vi "TalonSRXSetCoast.vi"(0 "Device Reference (in)":T1, 5 "Set Coast Mode":bool, 11 "Error (in)":errorcluster) -> (4 "Device Reference (out)":T1, 15 "Error (out)":errorcluster)   [LabVIEW 2020]
doc: "Wrapper for setting coast/brake mode for Talon SRX motor controllers."
uses:
  <vilib>/Rock Robotics/WPI/MotorControl/WPI_MotorControlDeviceRef.ctl
  <vilib>/Rock Robotics/WPI/MotorControl/WPI_MotorControlType.ctl
  <vilib>/Rock Robotics/SystemInterfaces/DIO/FPGA_DIOPWMChannel.ctl
  <vilib>/Rock Robotics/WPI/PWM/WPI_PWMDeadband.ctl
  <vilib>/Rock Robotics/SystemInterfaces/DIO/FPGA_DIOChannel.ctl
  <vilib>/Rock Robotics/WPI/ThirdParty/Phoenix-LabVIEW/Motor Controller/Controls/CTRE_Phoenix_MotorControl_NeutralMode.ctl
  3ee01901-79ae-4aa6-af32-efcf4cf19248.vi
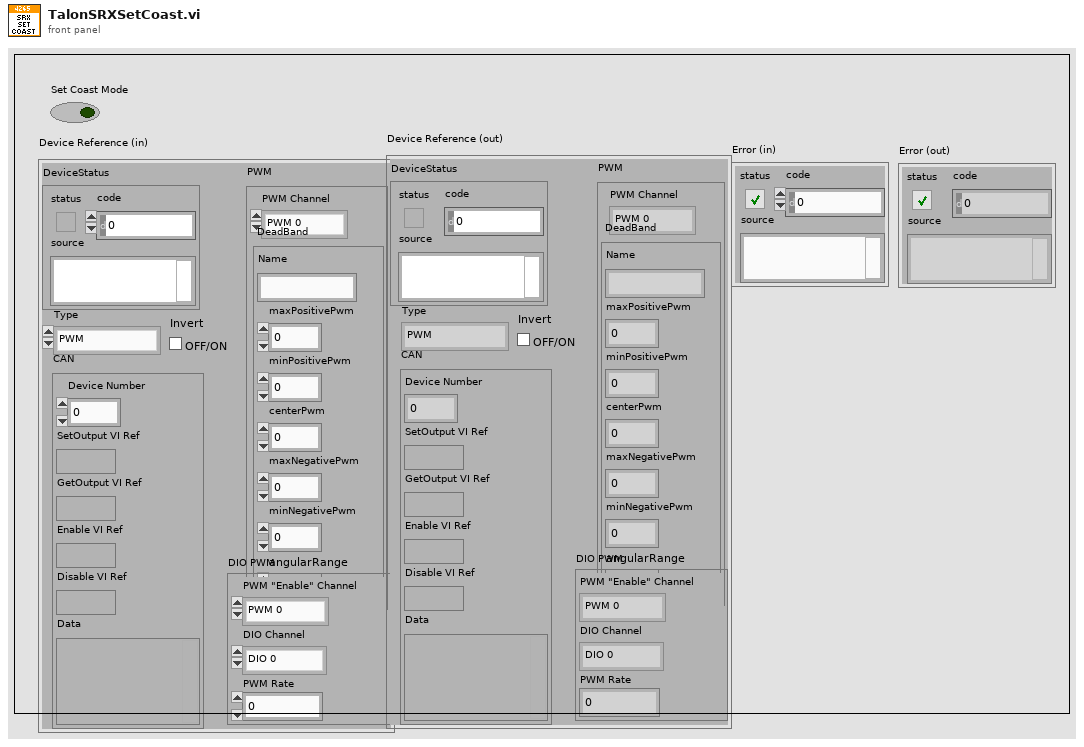
[diagram p1: front panel]
types:
  T1 = typedef "WPI_MotorControlDeviceRef.ctl" = cluster{"DeviceStatus":errorcluster, "Type":T2, "PWM":cluster{"PWM Channel":T3, "DeadBand":T4}, "CAN":cluster{"Device Number":u8, "SetOutput VI Ref":variant, "GetOutput VI Ref":variant, "Enable VI Ref":variant, "Disable VI Ref":variant, "Data":variant}, "Invert":bool, "DIO PWM":cluster{"PWM \"Enable\" Channel":T3, "DIOChannel":T5, "PWM Rate":dbl}}
  T2 = typedef "WPI_MotorControlType.ctl" = enum16{"PWM", "CAN", "DIO PWM"}
  T3 = typedef "FPGA_DIOPWMChannel.ctl" = enum8{"PWM 0", "PWM 1", "PWM 2", "PWM 3", "PWM 4", "PWM 5", "PWM 6", "PWM 7", "PWM 8", "PWM 9", "PWM MXP 0", "PWM MXP 1", "PWM MXP 2", "PWM MXP 3", "PWM MXP 4", "PWM MXP 5", "PWM MXP 6", "PWM MXP 7", "PWM MXP 8", "PWM MXP 9", "Invalid"}
  T4 = typedef "WPI_PWMDeadband.ctl" = cluster{"Name":string, "maxPositivePwm":i32, "minPositivePwm":i32, "centerPwm":i32, "maxNegativePwm":i32, "minNegativePwm":i32, "angularRange":u16}
  T5 = typedef "FPGA_DIOChannel.ctl" = enum8{"DIO 0", "DIO 1", "DIO 2", "DIO 3", "DIO 4", "DIO 5", "DIO 6", "DIO 7", "DIO 8", "DIO 9", "DIO MXP 0", "DIO MXP 1", "DIO MXP 2", "DIO MXP 3", "DIO MXP 4", "DIO MXP 5", "DIO MXP 6", "DIO MXP 7", "DIO MXP 8", "DIO MXP 9", "DIO MXP 10", "DIO MXP 11", "DIO MXP 12", "DIO MXP 13", "DIO MXP 14", "DIO MXP 15", "SPI Port CS1", "SPI Port CS2", "SPI Port CS3", "SPI Port MISO", "SPI Port MOSI", "Invalid"}
  T6 = typedef "CTRE_Phoenix_MotorControl_NeutralMode.ctl" = enum8{"EEPROMSetting", "Override to Coast", "Override to Brake"}
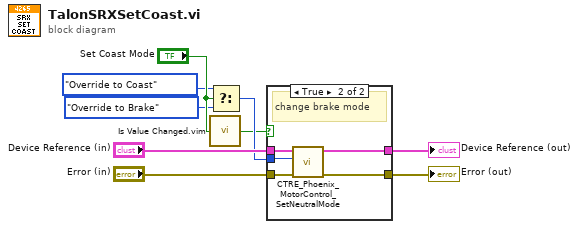
[diagram p0: block diagram]
diagram:
  n1 = call "Is Value Changed.vim"("value"="Set Coast Mode") -> ("changed or first call?"=w5:bool)
  n2 = Select(t=CTRE_Phoenix_MotorControl_NeutralMode."Override to Coast" ("Motor Control Neutral Mode"), s="Set Coast Mode", f=CTRE_Phoenix_MotorControl_NeutralMode."Override to Brake") -> (s? t:f=w6:T6)
  n3 = case shown="True" w5 {
    tunnel: "Device Reference (in)" -> [w11 w16]
    tunnel: [w11 w15] -> w1
    tunnel: "Error (in)" -> [w10 w14]
    tunnel: [w10 w13] -> w2
    tunnel: w6 -> [_ w12]
    frame False {
    }
    frame True {
      # "change brake mode"
      n4 = call <vilib>:"CTRE_Phoenix_MotorControl_SetNeutralMode.vi"("error in (no error)"=w14, "Motor Control Neutral Mode"=w12, "PhoenixMotorControlDevRef"=w16) -> ("error out"=w13:errorcluster, "PhoenixMotorControlDevRef"=w15:T1)  [unwired: 7 in]
    }
  }
  "Error (out)" <- w2
  "Device Reference (out)" <- w1
